vi "Encoder_SubVI_revised.vi"(0 "Velocity Interval (uSec)":fxp<+/-,40,24>=1000.0, 5 "A":bool=TRUE, 7 "B":bool=TRUE, 9 "Encoder Ticks Per Revolution":fxp<+/-,40,24>, 11 "Previous Variables Input":T1) -> (4 "Position (Degrees)":fxp<+/-,40,24>, 6 "Velocity (Degrees/Second)":fxp<+/-,40,24>, 15 "Previous Variables Output":T1)   [LabVIEW 2014]
uses:
  <vilib>/rvi/FXPMathLib/FxpDiv/subVIs/nifxpmath_Div_SimConfig.ctl
  <vilib>/rvi/FXPMathLib/FxpDiv/simVIs/DllFxpDivTemp_sub.vi
  <vilib>/rvi/FXPMathLib/FxpDiv/XNode/nifxpmath_Div.xnode
  <vilib>/rvi/FXPMathLib/FxpMul/XNode/nifxpmath_Multiplier.xnode
  <vilib>/rvi/FXPMathLib/sim/FxpSim.dll
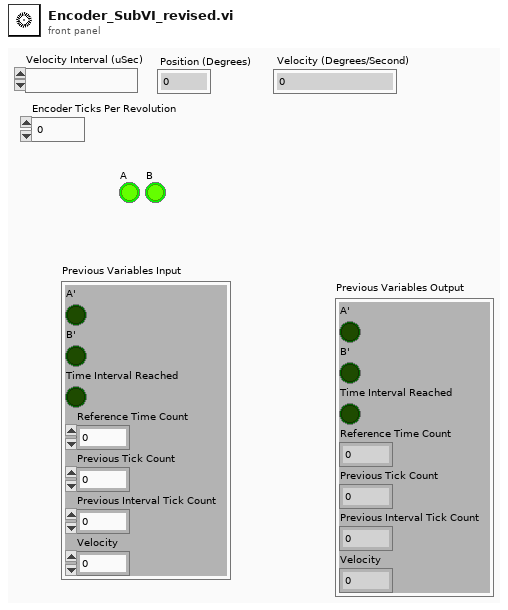
[diagram p1: front panel]
types:
  T1 = cluster{"A'":bool, "B'":bool, "Time Interval Reached":bool, "Reference Time Count":fxp<+/-,64,64>, "Previous Tick Count":fxp<+/-,40,24>, "Previous Interval Tick Count":fxp<+/-,40,24>, "Velocity":fxp<+/-,40,24>}
  T2 = cluster{"A":bool, "B":bool, bool, "Reference Time Count":fxp<+/-,64,64>, "Previous Tick Count":fxp<+/-,40,24>, "Previous Tick Count":fxp<+/-,40,24>, "Velocity":fxp<+/-,64,32>}
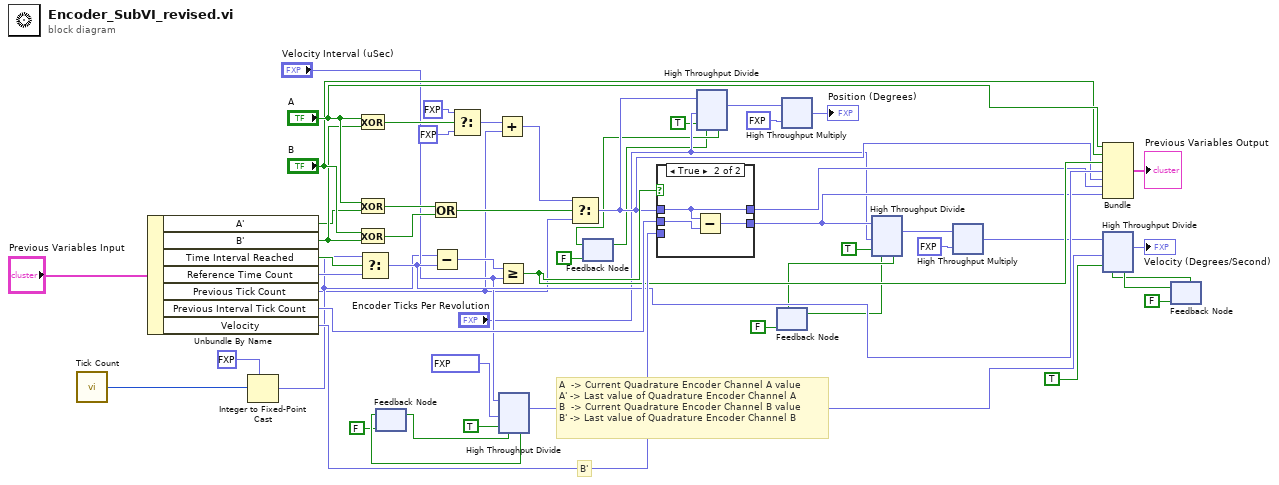
[diagram p0: block diagram]
diagram:
  # "A  -> Current Quadrature Encoder Channel A value\nA' -> Last value of Quadrature Encoder Channel A\nB  -> Current Quadrature Encoder Channel B value\nB' -> Last value of Quadrature Encoder Channel B"
  # "B'"
  n1 = call "Tick Count"() -> ("Tick Count(uSec)"=w28:u32)
  n2 = Unbundle By Name("Previous Variables Input") -> ("A'"=w35:bool, "B'"=w36:bool, "Time Interval Reached"=w54:bool, "Reference Time Count"=w53:fxp<+/-,64,64>, "Previous Tick Count"=w13:fxp<+/-,40,24>, "Previous Interval Tick Count"=w52:fxp<+/-,40,24>, "Velocity"=w51:fxp<+/-,40,24>)
  n3 = Integer to Fixed-Point Cast(fixed-point type=fxp<+/-,64,64> 0.0, integer=w28) -> (fixed-point=w26:fxp<+/-,64,64>)
  n4 = Exclusive Or(1:w36, 2:"A") -> (0:w38:bool)
  n5 = Exclusive Or(1:w35, 2:"A") -> (0:w39:bool)
  n6 = Exclusive Or(1:w36, 2:"B") -> (0:w40:bool)
  n7 = Select(t=w26, s=w54, f=w53) -> (s? t:f=w46:fxp<+/-,64,64>)
  n8 = feedback #1(FALSE ("ready for input")) -> (w10:bool)
  n9 = Or(x=w39, y=w40) -> (x .or. y?=w37:bool)
  n10 = Subtract(x=w26, y=w46) -> (x-y=w25:fxp<+/-,40,24>)
  n11 = Select(t=fxp<+/-,40,24> -1.0 ("32 bit"), s=w38, f=fxp<+/-,40,24> 1.0 ("32 bit")) -> (s? t:f=w43:fxp<+/-,40,24>)
  n12 = Add(x=w43, y=w13) -> (x+y=w44:fxp<+/-,40,24>)
  n13 = Greater Or Equal?(x=w25, y="Velocity Interval (uSec)") -> (x >= y?=w47:bool)
  n14 = xnode "High Throughput Divide"("x"="Velocity Interval (uSec)", "y"=fxp<+/-,40,24> 1000000.0 ("Velocity Interval (uSec)"), "input valid"=TRUE, "ready for output (T)"=w10) -> ("x/y"=w20:fxp<+/-,40,24>, "ready for input"=w12:bool)  [unwired: 1 out]
  n15 = feedback-in #1(w12) -> ()
  n16 = Select(t=w44, s=w37, f=w13) -> (s? t:f=w32:fxp<+/-,40,24>)
  n17 = feedback #2(FALSE ("ready for input")) -> (w2:bool)
  n18 = case shown="True" w47 {
    tunnel: w32 -> [_ w58]
    tunnel: w52 -> [w56 w60]
    tunnel: [w57 w59] -> w24
    tunnel: w51 -> [w57 _]
    tunnel: [w56 w58] -> w45
    frame False {
    }
    frame True {
      n19 = Subtract(x=w58, y=w60) -> (x-y=w59:fxp<+/-,64,32>)
    }
  }
  n20 = xnode "High Throughput Divide"("x"=w32, "y"="Encoder Ticks Per Revolution", "input valid"=TRUE, "ready for output (T)"=w2) -> ("x/y"=w31:fxp<+/-,40,24>, "ready for input"=w3:bool)  [unwired: 1 out]
  n21 = feedback-in #2(w3) -> ()
  n22 = feedback #3(FALSE ("ready for input")) -> (w5:bool)
  n23 = xnode ("High Throughput Multiply")("x"=w31, "y"=fxp<+/-,40,24> 360.0 ("Encoder Ticks Per Revolution")) -> ("x*y"=→"Position (Degrees)":fxp<+/-,40,24>)
  n24 = xnode "High Throughput Divide"("x"=w24, "y"="Encoder Ticks Per Revolution", "input valid"=TRUE, "ready for output (T)"=w5) -> ("x/y"=w21:fxp<+/-,40,24>, "ready for input"=w6:bool)  [unwired: 1 out]
  n25 = feedback-in #3(w6) -> ()
  n26 = xnode ("High Throughput Multiply")("x"=w21, "y"=fxp<+/-,40,24> 360.0 ("Velocity Interval (uSec)")) -> ("x*y"=w14:fxp<+/-,40,24>)
  n27 = Bundle("A"="A", "B"="B", w47, "Reference Time Count"=w46, "Previous Tick Count"=w32, "Previous Tick Count"=w45, "Velocity"=w24) -> (→"Previous Variables Output":T2)  [unwired: 1 in]
  n28 = feedback #4(FALSE ("ready for input")) -> (w8:bool)
  n29 = xnode "High Throughput Divide"("x"=w14, "y"=w20, "input valid"=TRUE, "ready for output (T)"=w8) -> ("x/y"=→"Velocity (Degrees/Second)":fxp<+/-,40,24>, "ready for input"=w9:bool)  [unwired: 1 out]
  n30 = feedback-in #4(w9) -> ()
